vi "StimulusProfile.RunAsynch.vi"(9 "uutSerialNumber":string, 10 "Stimulus Profile Path":string, 11 "gatewayIP":string) -> ()   [LabVIEW 2013, in "RTSequenceVIs.lvlib"]
uses:
  RTSequenceVIs.lvlib
  NationalInstruments.VeriStand.RealTimeSequenceDefinitionApi
panel:
  out "error out":errorcluster
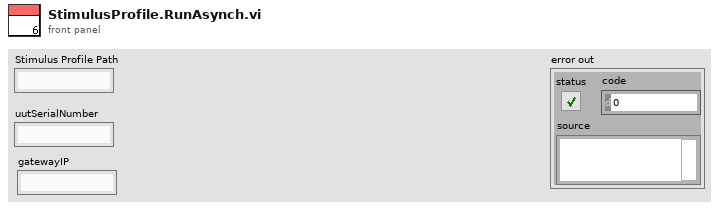
[diagram p1: front panel]
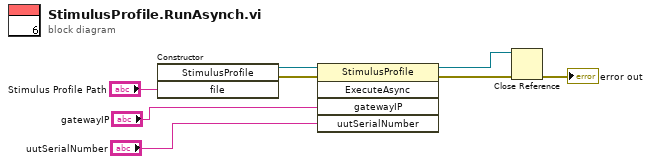
[diagram p0: block diagram]
diagram:
  n1 = constructor class="StimulusProfile"("file"="Stimulus Profile Path") -> (reference out=w8:refnum<k24>, error out=w7:errorcluster)  [unwired: 3 in, 2 out]
  n2 = invoke class="StimulusProfile" method="ExecuteAsync"(reference=w8, error in=w7, "gatewayIP"="gatewayIP", "uutSerialNumber"="uutSerialNumber") -> (reference out=w2:refnum<k24>, error out=w3:errorcluster)  [unwired: 1 in, 3 out]
  n3 = Close Reference(reference=w2, error in (no error)=w3) -> (error out=→"error out":errorcluster)
